vi "Output Subset.vi"(8 "error in (no error)":errorcluster, 10 "Output subset length":i32, 11 "Spectrum Recorder too in":refnum<class "Spectrum Recorder too.lvclass">) -> (0 "error out":errorcluster, 2 "Output subset":dbl[](array[numeric]), 3 "Spectrum Recorder too out":refnum<class "Spectrum Recorder too.lvclass">)   [LabVIEW 2024, in "Spectrum Recorder too.lvclass"]
uses:
  Spectrum Recorder too.lvclass
  Spectrum Recorder too.lvclass/Spectrum Recorder too.ctl
panel:
  out "x > y?":bool
  out "head  length":i32
  out "tail length":i32
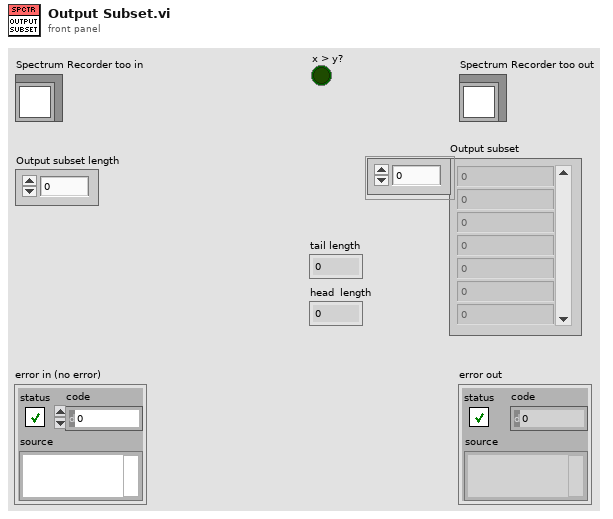
[diagram p1: front panel]
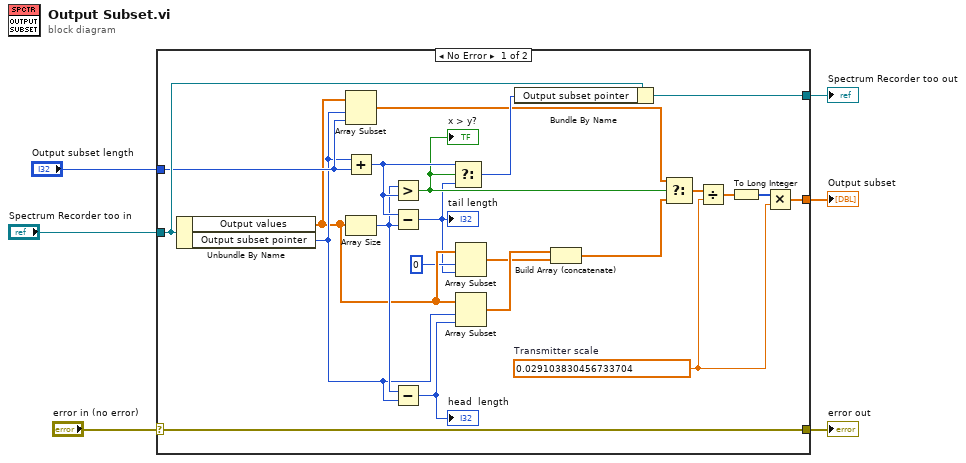
[diagram p0: block diagram]
diagram:
  n1 = case shown="No Error" "error in (no error)" {
    selector: "error in (no error)" -> [w28 w30]
    tunnel: [w28 w30] -> w5
    tunnel: [w26 w29] -> w3
    tunnel: "Spectrum Recorder too in" -> [w27 w29]
    tunnel: "Output subset length" -> [w23 _]
    tunnel: [w7 _] -> w1
    frame No Error {
      w9 = 0.029103830456733704  # Transmitter scale
      n2 = Unbundle By Name(w27) -> ("Output values"=w17:dbl[], "Output subset pointer"=w19:i32)
      n3 = Array Subset(array=w17, index=w19, length=w23) -> (w21:dbl[])
      n4 = Add(x=w19, y=w23) -> (x+y=w24:i32)
      n5 = Array Size(array=w17) -> (size(s)=w20:i32)
      n6 = Greater?(x=w20, y=w24) -> (0:w22:bool)
      "x > y?" <- w22
      n7 = Subtract(x=w24, y=w20) -> (x-y=w12:i32)
      "tail length" <- w12
      n8 = Subtract(x=w20, y=w19) -> (x-y=w18:i32)
      "head  length" <- w18
      n9 = Select(t=w24, s=w22, f=w12) -> (s? t:f=w25:i32)
      n10 = Array Subset(array=w17, index=0, length=w12) -> (w14:dbl[])
      n11 = Array Subset(array=w17, index=w19, length=w18) -> (w15:dbl[])
      n12 = Bundle By Name(cluster=w27, "Output subset pointer"=w25) -> (w26:refnum<class "Spectrum Recorder too.lvclass">)
      n13 = Build Array (concatenate)(w15, w14) -> (w13:dbl[])
      n14 = Select(t=w21, s=w22, f=w13) -> (s? t:f=w8:dbl[])
      n15 = Divide(x=w8, y=w9) -> (x/y=w11:dbl[])
      n16 = To Long Integer(number=w11) -> (32bit integer=w10:i32[])
      n17 = Multiply(x=w10, y=w9) -> (x*y=w7:dbl[])
    }
    frame Error {
    }
  }
  "error out" <- w5
  "Spectrum Recorder too out" <- w3
  "Output subset" <- w1
